vi "FromMatlabParam.vi"(4 "Allow Variant Values (f)":bool, 10 "Matlab Param Data":T1[](array[typedef]), 11 "Type (or value to update)":variant) -> (3 "Value":variant)   [LabVIEW 2017]
uses:
  LVPort/Matlab/VI/ObjectMap/LVPortMatlabNamepathData2.ctl
  LVPort/Matlab/VI/ObjectMap/LVPortMatlabDataTypeEnum_2.ctl
  LVPort/Matlab/VI/ObjectMap/LVPortMatlabContainerTypeEnum_2.ctl
panel:
  out "Conversion messages":string[](array[string])
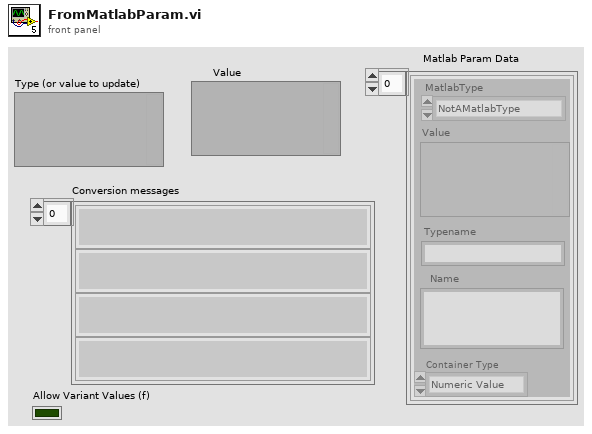
[diagram p1: front panel]
types:
  T1 = typedef "LVPortMatlabNamepathData2.ctl" = cluster{"MatlabType":T2, "Value":variant, "Name":string, "Typename":string, "Container Type":T3}
  T2 = typedef "LVPortMatlabDataTypeEnum_2.ctl" = enum16{"NotAMatlabType", "Real", "Complex", "String", "Boolean"}
  T3 = typedef "LVPortMatlabContainerTypeEnum_2.ctl" = enum16{"Numeric Value", "Numeric Array", "Waveform"}
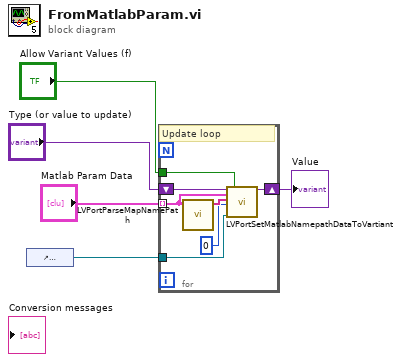
[diagram p0: block diagram]
diagram:
  n1 = control-ref of="Conversion messages"() -> (w2:refnum<vi>)
  n2 = for {
    tunnel: "Matlab Param Data" -> [w8] mode=indexing
    shift-right: [w10] -> w4
    shift-left: "Type (or value to update)" -> [w11]
    tunnel: w2 -> [w7]
    tunnel: "Allow Variant Values (f)" -> [w6]
    # "Update loop"
    n3 = call "LVPortParseMapNamePath.vi"("MatlabDataBundle"=w8) -> ("Name parts array"=w12:string[])  [unwired: 10 in]
    n4 = call "LVPortSetMatlabNamepathDataToVartiant.vi"("Type (or value to update)"=w11, "MatlabDataBundle"=w8, "NamePath"=w12, "Namepath Index"=0 ("curNameIndex"), "Info collection refrence in"=w7, "Allow Variant Values (f)"=w6) -> ("Value"=w10:variant)  [unwired: 12 in, 1 out]
  }
  "Value" <- w4
